vi "MB_SwerveOdometry_UpdateX.vi"(8 "module Positions":T6[](array[typedef]) {"Angle"."SIN" format="%13.4f"; "Angle"."COS" format="%13.4f"; "Angle"."VALUE" format="%13.4f"}, 9 "gyroAngle":T5={"VALUE"=0.0, "COS"=1.0, "SIN"=0.0} {"SIN" format="%13.4f"; "COS" format="%13.4f"; "VALUE" format="%13.4f"}, 10 "in SWERVE_DRIVE_ODOMETRY":T8={"POSE"={"TRANSLATION"={"X"=0.0, "Y"=0.0}, "ROTATION"={"VALUE"=0.0, "COS"=1.0, "SIN"=0.0}}, "GyroOffset"={"VALUE"=0.0, "COS"=1.0, "SIN"=0.0}, "PreviousAngle"={"VALUE"=0.0, "COS"=1.0, "SIN"=0.0}, "PrevModulePositions"=[], "NumModules"=0} {"PrevModulePositions"."Angle"."SIN" format="%13.4f"; "PrevModulePositions"."Angle"."COS" format="%13.4f"; "PrevModulePositions"."Angle"."VALUE" format="%13.4f"; "PreviousAngle"."SIN" format="%13.4f"; "PreviousAngle"."COS" format="%13.4f"; "PreviousAngle"."VALUE" format="%13.4f"; "GyroOffset"."SIN" format="%13.4f"; "GyroOffset"."COS" format="%13.4f"; "GyroOffset"."VALUE" format="%13.4f"; "POSE"."ROTATION"."SIN" format="%13.4f"; "POSE"."ROTATION"."COS" format="%13.4f"; "POSE"."ROTATION"."VALUE" format="%13.4f"; "POSE"."TRANSLATION"."Y" format="%14.3f"; "POSE"."TRANSLATION"."X" format="%14.3f"}, 11 "SWERVE_DRIVE_KINEMATICS":T1 {"SavedModuleStates"."Angle"."SIN" format="%13.4f"; "SavedModuleStates"."Angle"."COS" format="%13.4f"; "SavedModuleStates"."Angle"."VALUE" format="%13.4f"; "PrevCoR"."Y" format="%14.3f"; "PrevCoR"."X" format="%14.3f"; "Modules"."Y" format="%14.3f"; "Modules"."X" format="%14.3f"}) -> (0 "Error":bool, 1 "robot POSE":T7={"TRANSLATION"={"X"=0.0, "Y"=0.0}, "ROTATION"={"VALUE"=0.0, "COS"=1.0, "SIN"=0.0}} {"ROTATION"."SIN" format="%13.4f"; "ROTATION"."COS" format="%13.4f"; "ROTATION"."VALUE" format="%13.4f"; "TRANSLATION"."Y" format="%14.3f"; "TRANSLATION"."X" format="%14.3f"}, 3 "out SWERVE_DRIVE_ODOMETRY":T8={"POSE"={"TRANSLATION"={"X"=0.0, "Y"=0.0}, "ROTATION"={"VALUE"=0.0, "COS"=1.0, "SIN"=0.0}}, "GyroOffset"={"VALUE"=0.0, "COS"=1.0, "SIN"=0.0}, "PreviousAngle"={"VALUE"=0.0, "COS"=1.0, "SIN"=0.0}, "PrevModulePositions"=[], "NumModules"=0} {"PrevModulePositions"."Angle"."SIN" format="%13.4f"; "PrevModulePositions"."Angle"."COS" format="%13.4f"; "PrevModulePositions"."Angle"."VALUE" format="%13.4f"; "PreviousAngle"."SIN" format="%13.4f"; "PreviousAngle"."COS" format="%13.4f"; "PreviousAngle"."VALUE" format="%13.4f"; "GyroOffset"."SIN" format="%13.4f"; "GyroOffset"."COS" format="%13.4f"; "GyroOffset"."VALUE" format="%13.4f"; "POSE"."ROTATION"."SIN" format="%13.4f"; "POSE"."ROTATION"."COS" format="%13.4f"; "POSE"."ROTATION"."VALUE" format="%13.4f"; "POSE"."TRANSLATION"."Y" format="%14.3f"; "POSE"."TRANSLATION"."X" format="%14.3f"})   [LabVIEW 2020]
doc: "Updates the robot's position on the field using forward kinematics and integration of the pose over time. This method takes in the current time as a parameter to calculate period (difference between two timestamps). The period is used to calculate the change in distance from a velocity. Thisalso takes in an angle parameter which is used instead of the angular rate that is calculated from forward kinematics.\n\nParameters:\n - InSwerveDriveKinematics - The data structure \n - InSwerveDriveOdometry - This data structure \n - gyroAngle - The angle reported by the gyroscope.\n - modulePositions - The current positions (distances) of all swerve modules. Please provide the states in the same order in which you instantiated your SwerveDriveKinematics.\n\nReturns:\n - OutSwerveDriveOdometry - Updated data structure\n - The new pose of the robot.\n - Error -- TRUE if an error occured (number of modules doesn't match)"
uses:
  <vilib>/Rock Robotics/WPI/ThirdParty/JAS_Junk/TrajLib/TypeDef/ROTATION2D.ctl
  <vilib>/Rock Robotics/WPI/ThirdParty/JAS_Junk/TrajLib/TypeDef/SWERVE_DRIVE_ODOMETRY.ctl
  <vilib>/Rock Robotics/WPI/ThirdParty/JAS_Junk/TrajLib/TypeDef/POSE2D.ctl
  <vilib>/Rock Robotics/WPI/ThirdParty/JAS_Junk/TrajLib/TypeDef/TRANSLATION2D.ctl
  <vilib>/Rock Robotics/WPI/ThirdParty/JAS_Junk/TrajLib/TypeDef/SWERVE_DRIVE_MODULE_POSITION.ctl
  <vilib>/Rock Robotics/WPI/ThirdParty/JAS_Junk/TrajLib/TypeDef/SWERVE_DRIVE_KINEMATICS.ctl
  <vilib>/Analysis/Matrix/Datatypes/RealMatrix.ctl
  <vilib>/Rock Robotics/WPI/ThirdParty/JAS_Junk/TrajLib/TypeDef/SWERVE_DRIVE_MODULE_STATE.ctl
  <vilib>/Rock Robotics/WPI/ThirdParty/JAS_Junk/TrajLib/Rotation2d_CreateXY.vi
  <vilib>/Rock Robotics/WPI/ThirdParty/JAS_Junk/TrajLib/Rotation2d_CreateAngle.vi
  <vilib>/Rock Robotics/WPI/ThirdParty/JAS_Junk/TrajLib/Util_CalcDist.vi
  <vilib>/Rock Robotics/WPI/ThirdParty/JAS_Junk/TrajLib/Trajectory_Library.lvlib
  <vilib>/Rock Robotics/WPI/ThirdParty/JAS_Junk/TrajLib/TypeDef/TWIST2D.ctl
  <vilib>/Analysis/Matrix/NI_Matrix.lvlib
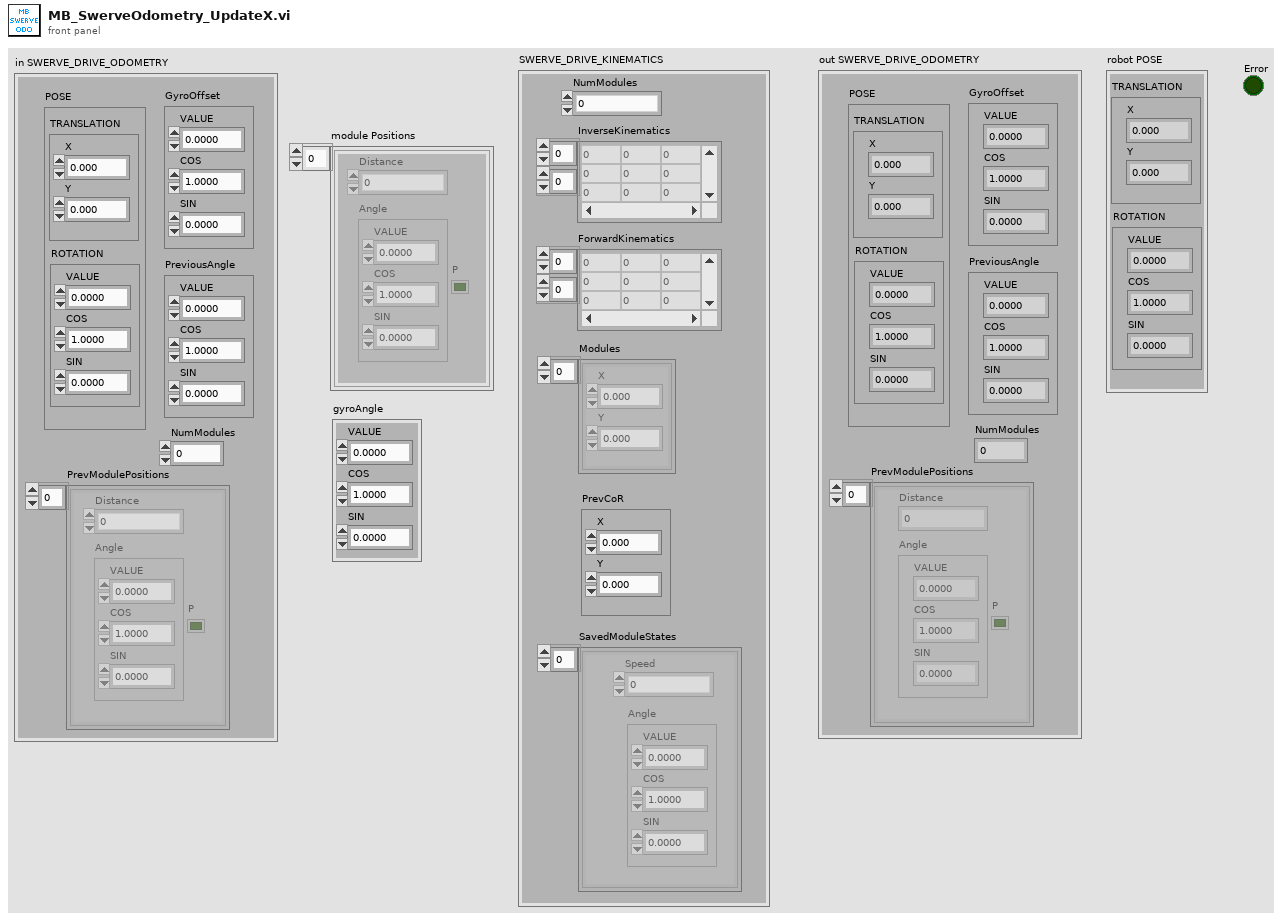
[diagram p1: front panel]
types:
  T1 = typedef "Trajectory_Library.lvlib/SWERVE_DRIVE_KINEMATICS.ctl" = cluster{"NumModules":i32, "InverseKinematics":T2, "ForwardKinematics":T2, "Modules":T3[], "PrevCoR":T3, "SavedModuleStates":T4[]}
  T2 = typedef "NI_Matrix.lvlib/RealMatrix.ctl" = dbl[][]
  T3 = typedef "Trajectory_Library.lvlib/TRANSLATION2D.ctl" = cluster{"X":dbl, "Y":dbl}
  T4 = typedef "Trajectory_Library.lvlib/SWERVE_DRIVE_MODULE_STATE.ctl" = cluster{"Speed":dbl, "Angle":T5}
  T5 = typedef "Trajectory_Library.lvlib/ROTATION2D.ctl" = cluster{"VALUE":dbl, "COS":dbl, "SIN":dbl}
  T6 = typedef "Trajectory_Library.lvlib/SWERVE_DRIVE_MODULE_POSITION.ctl" = cluster{"Distance":dbl, "Angle":T5, "P":bool}
  T7 = typedef "Trajectory_Library.lvlib/POSE2D.ctl" = cluster{"TRANSLATION":T3, "ROTATION":T5}
  T8 = typedef "Trajectory_Library.lvlib/SWERVE_DRIVE_ODOMETRY.ctl" = cluster{"POSE":T7, "GyroOffset":T5, "PreviousAngle":T5, "PrevModulePositions":T6[], "NumModules":i32}
  T9 = typedef "Trajectory_Library.lvlib/TWIST2D.ctl" = cluster{"dX":dbl, "dY":dbl, "dTHETA":dbl}
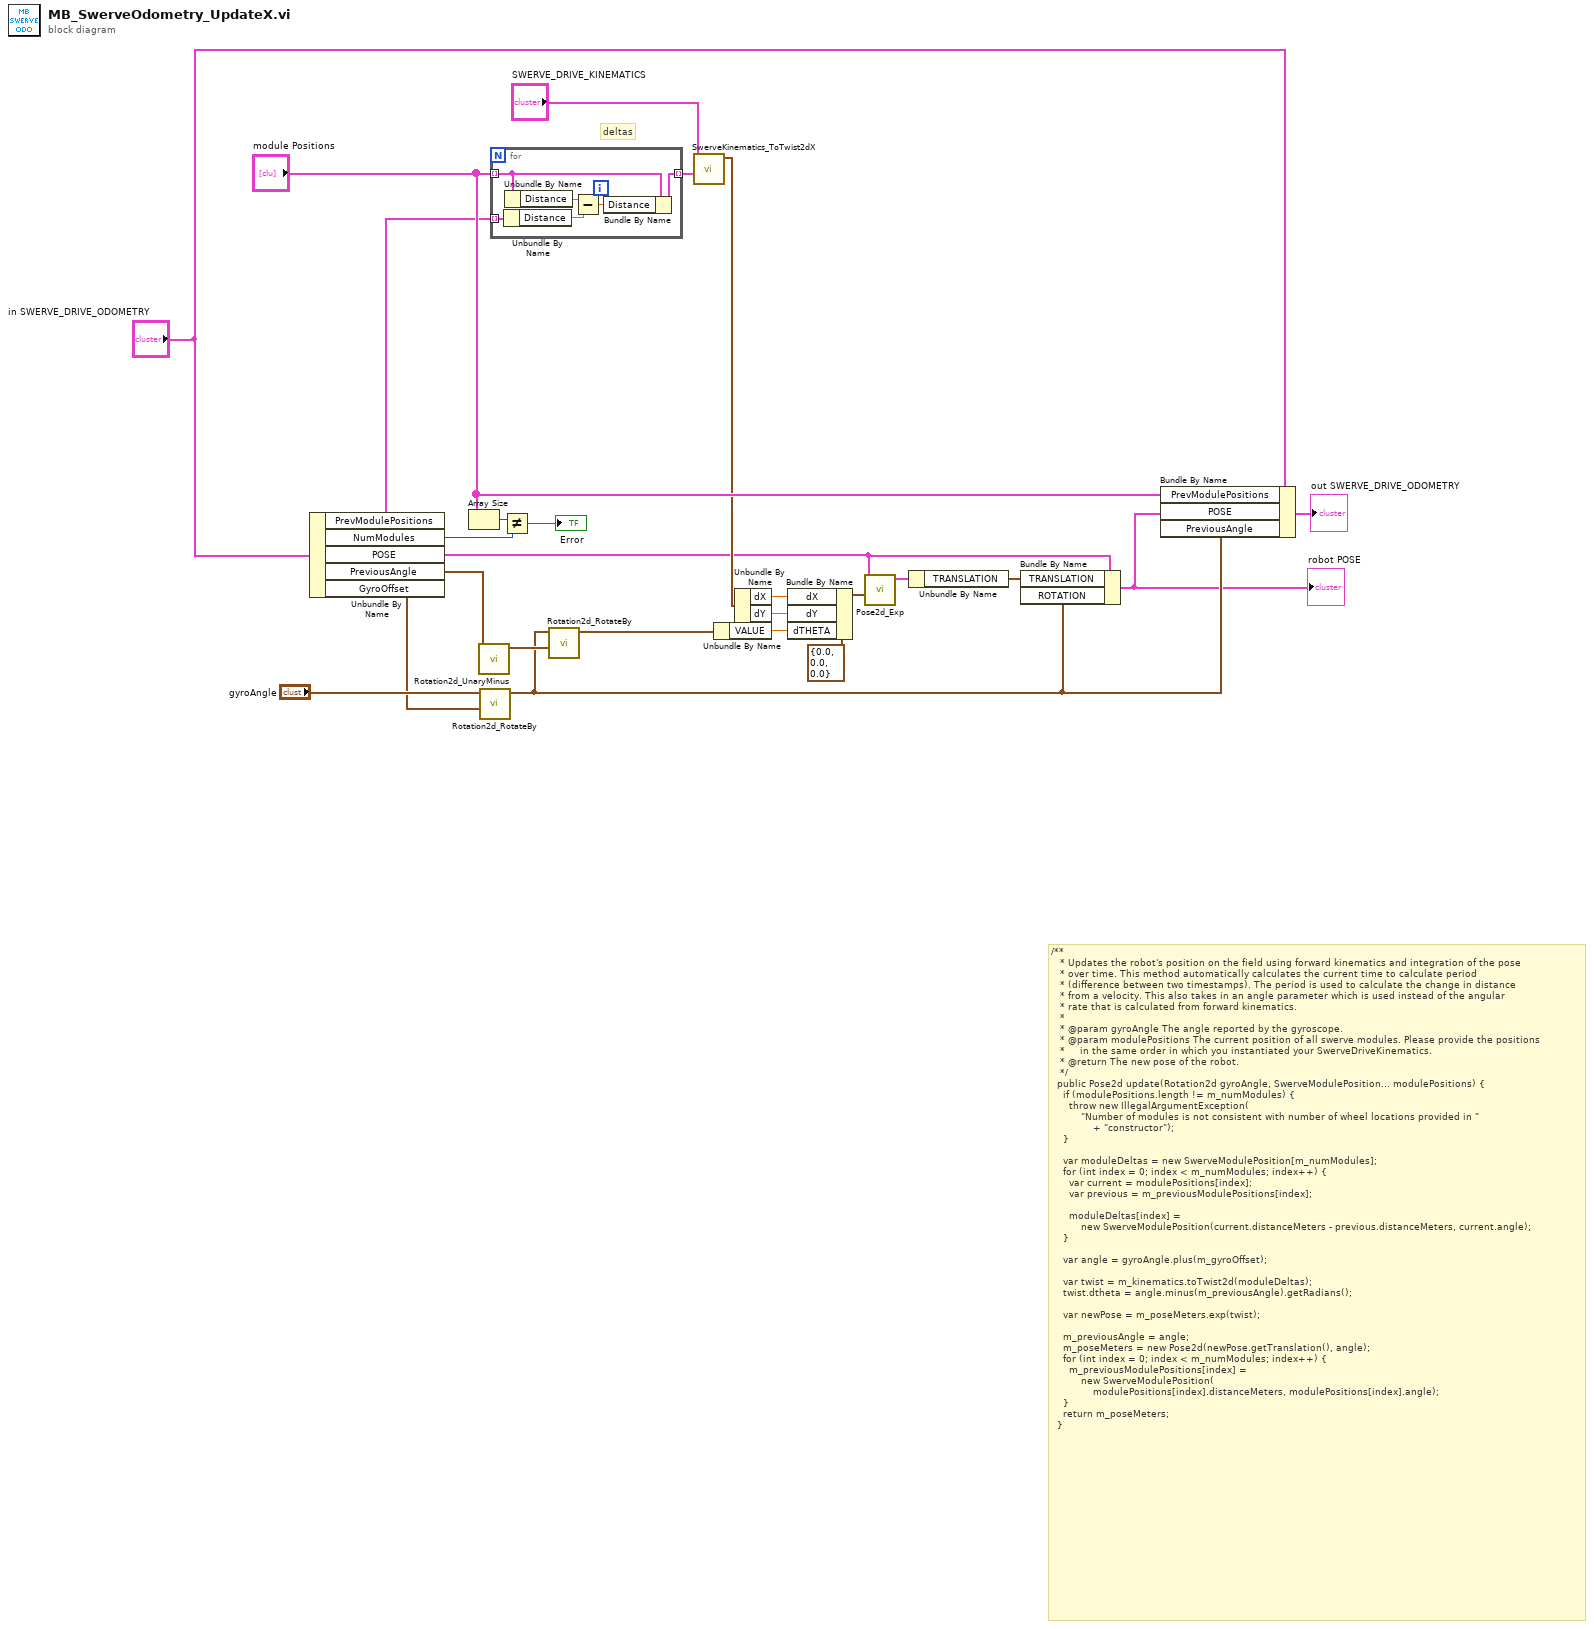
[diagram p0: block diagram]
diagram:
  # "deltas"
  # "/**\n   * Updates the robot's position on the field using forward kinematics and integration of the pose\n   * over time. This method automatically calculates the current time to calculate period\n   * (difference between two timestamps). The period is used to calculate the change in distance\n   * from a velocity. This also takes in an angle parameter which is used instead of the angular\n   * rate that is calculated from forward kinematics.\n   *\n   * @param gyroAngle The angle reported by the gyroscope.\n   * @param modulePositions The current position of all swerve modules. Please provide the positions\n   *     in the same order in which you instantiated your SwerveDriveKinematics.\n   * @return The new pose of the robot.\n   */\n  public Pose2d update(Rotation2d gyroAngle, SwerveModulePosition... modulePositions) {\n    if (modulePositions.length != m_numModules) {\n      throw new IllegalArgumentException(\n          \"Number of modules is not consistent with number of wheel locations provided in \"\n              + \"constructor\");\n    }\n\n    var moduleDeltas = new SwerveModulePosition[m_numModules];\n    for (int index = 0; index < m_numModules; index++) {\n      var current = modulePositions[index];\n      var previous = m_previousModulePositions[index];\n\n      moduleDeltas[index] =\n          new SwerveModulePosition(current.distanceMeters - previous.distanceMeters, current.angle);\n    }\n\n    var angle = gyroAngle.plus(m_gyroOffset);\n\n    var twist = m_kinematics.toTwist2d(moduleDeltas);\n    twist.dtheta = angle.minus(m_previousAngle).getRadians();\n\n    var newPose = m_poseMeters.exp(twist);\n\n    m_previousAngle = angle;\n    m_poseMeters = new Pose2d(newPose.getTranslation(), angle);\n    for (int index = 0; index < m_numModules; index++) {\n      m_previousModulePositions[index] =\n          new SwerveModulePosition(\n              modulePositions[index].distanceMeters, modulePositions[index].angle);\n    }\n    return m_poseMeters;\n  }"
  n1 = Unbundle By Name("in SWERVE_DRIVE_ODOMETRY") -> ("PrevModulePositions"=w7:T6[], "NumModules"=w22:i32, "POSE"=w4:T7, "PreviousAngle"=w8:T5, "GyroOffset"=w6:T5)
  n2 = Array Size(array="module Positions") -> (size(s)=w23:i32)
  n3 = call <vilib>:"Rotation2d_UnaryMinus.vi"("in ROTATION"=w8) -> ("out ROTATION"=w15:T5)  [unwired: 10 in]
  n4 = call <vilib>:"Rotation2d_RotateBy.vi"("other Rotation"=w6, "in ROTATION"="gyroAngle") -> ("out ROTATION"=w3:T5)  [unwired: 9 in]
  n5 = for {
    tunnel: w7 -> [w30] mode=indexing
    tunnel: "module Positions" -> [w28] mode=indexing
    tunnel: [w27] -> w19 mode=indexing
    n6 = Unbundle By Name(w30) -> ("Distance"=w29:dbl)
    n7 = Unbundle By Name(w28) -> ("Distance"=w31:dbl)
    n8 = Subtract(x=w31, y=w29) -> (x-y=w26:dbl)
    n9 = Bundle By Name(cluster=w28, "Distance"=w26) -> (w27:T6)
  }
  n10 = Not Equal?(x=w23, y=w22) -> (x != y?=→"Error":bool)
  n11 = call <vilib>:"Rotation2d_RotateBy.vi"("other Rotation"=w15, "in ROTATION"=w3) -> ("out ROTATION"=w14:T5)  [unwired: 9 in]
  n12 = call <vilib>:"SwerveKinematics_ToTwist2dX.vi"("WheelDeltas"=w19, "in SWERVE_DRIVE_KINEMATICS"="SWERVE_DRIVE_KINEMATICS") -> ("Twist2d"=w17:T9)  [unwired: 8 in, 1 out]
  n13 = Unbundle By Name(w14) -> ("VALUE"=w9:dbl)
  n14 = Unbundle By Name(w17) -> ("dX"=w11:dbl, "dY"=w10:dbl)
  n15 = Bundle By Name(cluster=T9 {"dX"=0.0, "dY"=0.0, "dTHETA"=0.0} ("TWIST"), "dX"=w11, "dY"=w10, "dTHETA"=w9) -> (w12:T9)
  n16 = call <vilib>:"Pose2d_Exp.vi"("TWIST"=w12, "POSE"=w4) -> ("UpdatedPose"=w5:T7)  [unwired: 9 in]
  n17 = Unbundle By Name(w5) -> ("TRANSLATION"=w2:T3)
  n18 = Bundle By Name(cluster=w4, "TRANSLATION"=w2, "ROTATION"=w3) -> (w1:T7)
  "robot POSE" <- w1
  n19 = Bundle By Name(cluster="in SWERVE_DRIVE_ODOMETRY", "PrevModulePositions"="module Positions", "POSE"=w1, "PreviousAngle"=w3) -> (→"out SWERVE_DRIVE_ODOMETRY":T8)
